vi "init.vi"(8 "error in (no error)":errorcluster, 11 "ESP300 in":refnum<class "ESP300.lvclass">) -> (0 "error out":errorcluster, 3 "ESP300 out":refnum<class "ESP300.lvclass">)   [LabVIEW 2018, in "ESP300.lvclass"]
uses:
  ESP300.lvclass
  _delayStageBase/_delayStageBase.lvclass
panel:
  out "resource name out":string
  in  "resource name":string
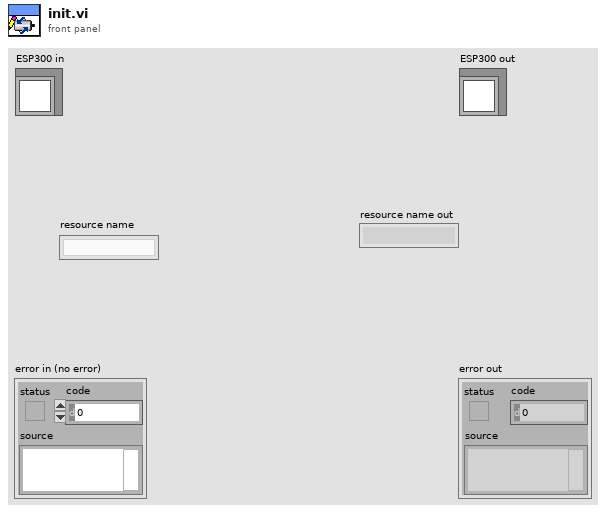
[diagram p1: front panel]
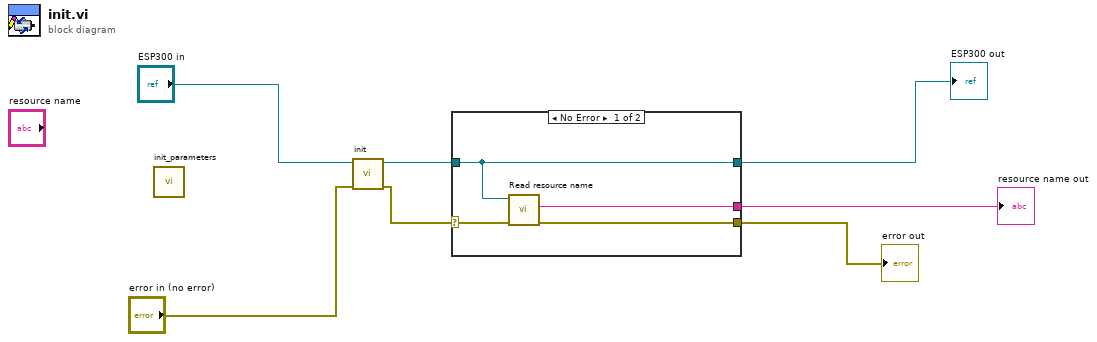
[diagram p0: block diagram]
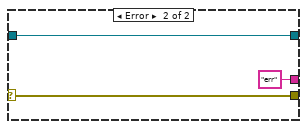
[diagram p2: hidden frame]
diagram:
  n1 = call "init_parameters.vi"() -> ()  [unwired: 11 in, 1 out]
  n2 = call-parent "init.vi"("error in (no error)"="error in (no error)", "_delayStageBase in"="ESP300 in") -> ("error out"=w1:errorcluster, "_delayStageBase out"=w5:refnum<class "ESP300.lvclass">)  [unwired: 8 in]
  n3 = case shown="No Error" w1 {
    selector: w1 -> [w10 w14]
    tunnel: [w9 w14] -> w3
    tunnel: w5 -> [w11 w13]
    tunnel: [w11 w13] -> w4
    tunnel: [w8 "err" ("resource name")] -> w2
    frame No Error {
      n4 = call-dynamic "Read resource name.vi"("error in (no error)"=w10, "_delayStageBase in"=w11) -> ("error out"=w9:errorcluster, "resource name"=w8:string)  [unwired: 7 in, 1 out]
    }
    frame Error {
    }
  }
  "error out" <- w3
  "ESP300 out" <- w4
  "resource name out" <- w2
